vi "Read Packet.vi"(8 "error in (no error)":errorcluster, 10 "capture_data_buffer":string, 11 "pcap reference":u64) -> (0 "error out":errorcluster, 2 "capture_data out":string, 3 "pcap reference out":u64, 4 "timeout":bool, 5 "Total Length":u32, 6 "EOF":bool, 7 "timestamp_seconds":dbl)   [LabVIEW 2025, in "Automotive Ethernet Bus Monitor UI.lvlib" / "lvwpcap.lvlib"]
doc: "This VI reads an ethernet packet. It outputs the packet in the form of a raw string."
uses:
  lvwpcap.lvlib
  lvwpcap.dll
panel:
  # "Select Help»Show Context Help and move the cursor over the VI icon to display help for this VI."
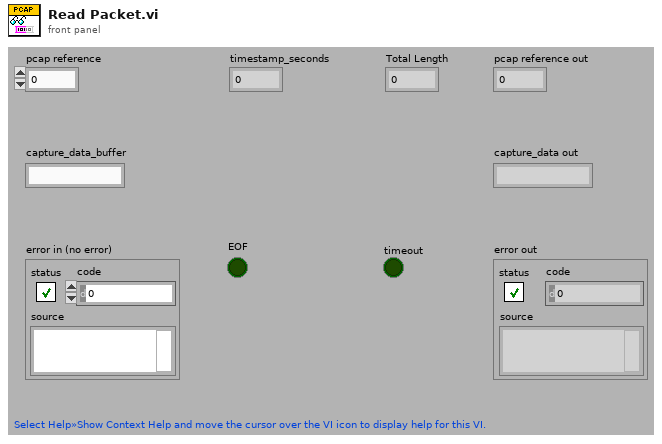
[diagram p1: front panel]
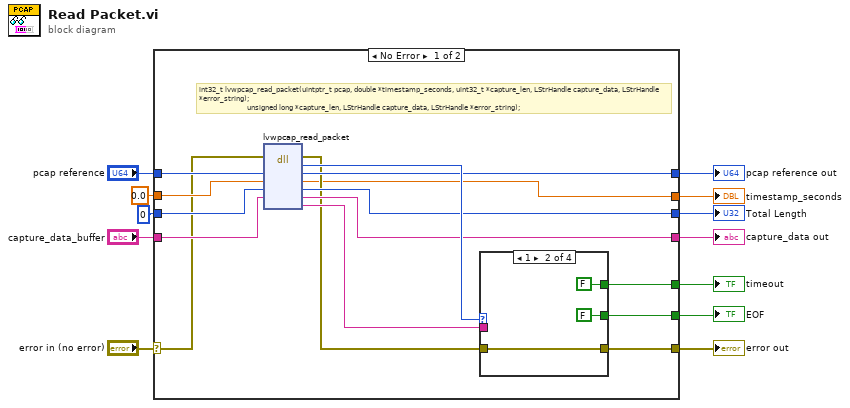
[diagram p0: block diagram]
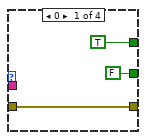
[diagram p2: hidden frame]
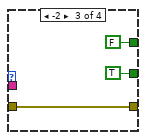
[diagram p3: hidden frame]
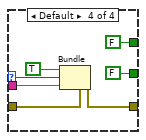
[diagram p4: hidden frame]
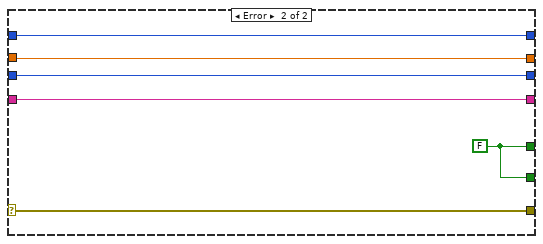
[diagram p5: hidden frame]
diagram:
  n1 = case shown="No Error" "error in (no error)" {
    selector: "error in (no error)" -> [w15 w49]
    tunnel: [w27 w49] -> w12
    tunnel: [w24 w46] -> w10
    tunnel: "pcap reference" -> [w23 w48]
    tunnel: 0.0 ("tv_sec (dummy)") -> [w22 w44]
    tunnel: u32 0 ("capture_len (dummy)") -> [w21 w45]
    tunnel: "capture_data_buffer" -> [w20 w47]
    tunnel: [w19 w48] -> w5
    tunnel: [w18 w45] -> w1
    tunnel: [w17 w47] -> w4
    tunnel: [w14 w46] -> w3
    tunnel: [w13 w44] -> w2
    frame No Error {
      # "int32_t lvwpcap_read_packet(uintptr_t pcap, double *timestamp_seconds, uint32_t *capture_len, LStrHandle capture_data, LStrHandle *error_string);\n                        unsigned long *capture_len, LStrHandle capture_data, LStrHandle *error_string);"
      n2 = dll-call lib="lvwpcap.dll" fn="lvwpcap_read_packet"(error in=w15, "pcap"=w23, "timestamp_seconds"=w22, "capture_len"=w21, "capture_data"=w20) -> (error out=w16:errorcluster, "return type"=w26:i32, "pcap"=w19:u64, "timestamp_seconds"=w13:dbl, "capture_len"=w18:u32, "capture_data"=w17:string, "error_string"=w25:string)  [unwired: 3 in, 1 out]
      n3 = case shown="1" w26 {
        selector: w26 -> [_ _ _ w42]
        tunnel: w25 -> [_ _ _ w41]
        tunnel: w16 -> [w30 w33 w35 w43]
        tunnel: [w30 w33 w35 w39] -> w27
        tunnel: [TRUE FALSE FALSE FALSE] -> w24
        tunnel: [FALSE FALSE TRUE FALSE] -> w14
        frame 0 {
        }
        frame 1 {
        }
        frame -2 {
        }
        frame Default {
          n4 = Bundle(cluster=w43, "status"=TRUE, "code"=w42, "source"=w41) -> (w39:errorcluster)
        }
      }
    }
    frame Error {
      w46 = FALSE
    }
  }
  "error out" <- w12
  "timeout" <- w10
  "pcap reference out" <- w5
  "capture_data out" <- w4
  "EOF" <- w3
  "timestamp_seconds" <- w2
  "Total Length" <- w1
